vi "LoggerDisable.vi"(8 "error in (no error)":errorcluster, 11 "LoggingActor in":refnum<class "LoggingActor.lvclass">) -> (0 "error out":errorcluster, 3 "LoggingActor out":refnum<class "LoggingActor.lvclass">)   [LabVIEW 2022 SP3, in "LoggingActor.lvlib" / "LoggingActor.lvclass"]
uses:
  LoggingActor.lvclass
  LoggingActor.lvclass/LoggingActor.ctl
  Logger/Source/Logger/Logger.lvclass
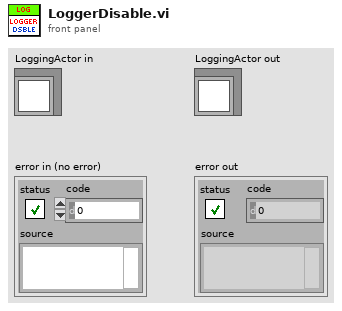
[diagram p1: front panel]
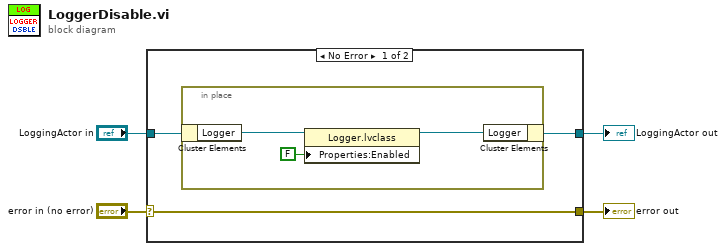
[diagram p0: block diagram]
diagram:
  n1 = case shown="No Error" "error in (no error)" {
    selector: "error in (no error)" -> [w7 w12]
    tunnel: [w7 w12] -> w3
    tunnel: [w5 w11] -> w1
    tunnel: "LoggingActor in" -> [w6 w11]
    frame No Error {
      n2 = in-place {
        n3 = in-place-cluster #1(w6) -> ("Logger"=w10:refnum<class "Logger.lvclass">)
        n4 = property class="Logger.lvclass"(reference=w10, "Properties:Enabled"=FALSE ("Enabled")) -> (reference out=w9:refnum<class "Logger.lvclass">)  [unwired: 1 in, 1 out]
        n5 = in-place-cluster #1("Logger"=w9) -> (w5:refnum<class "LoggingActor.lvclass">)
      }
    }
    frame Error {
    }
  }
  "error out" <- w3
  "LoggingActor out" <- w1
